vi "ChooseZones.vi"(8 "error in (no error)":errorcluster, 9 "NumberOfAttackers":i32, 10 "Game":refnum<class "Game.lvclass">, 11 "object in":refnum<class "Ally.lvclass">) -> (0 "error out":errorcluster, 2 "Zones":refnum<class "Zone.lvclass">[](array[class]), 3 "object out":refnum<class "Ally.lvclass">)   [LabVIEW 2023, in "Ally.lvclass"]
uses:
  Ally.lvclass
  Game_class/Game.lvclass
  Zone_class/Zone.lvclass
  Ally.lvclass/Ally.ctl
  Game_class/Game.lvclass/Game.ctl
  Parameters_class/Parameters.lvclass/Parameters.ctl
  Zone_class/zones.ctl
  Game_class/Read FieldRef.vi
  Game_class/Read NewParameters.vi
  Game_class/Read Parameters.lvclass.vi
  Parameters_class/Read AttakingOurselves.vi
  Field_class/Field.lvclass
  Parameters_class/Parameters.lvclass
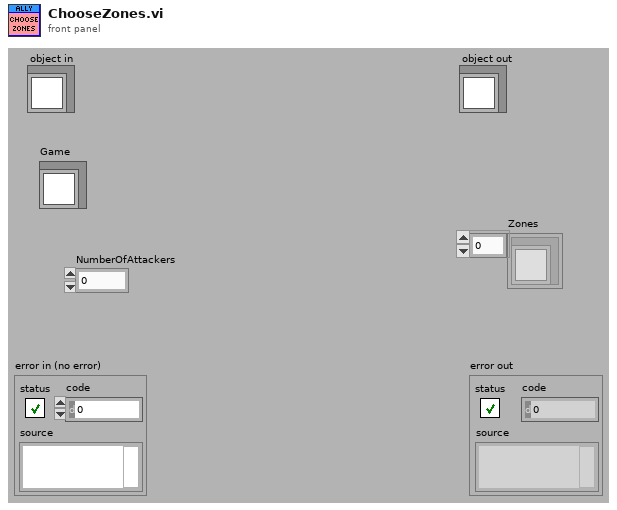
[diagram p1: front panel]
types:
  T1 = typedef "NewParameters.ctl" = cluster{"PenaltyDistance":dbl, "DistanceAttackerToBackBall":dbl, "Division":enum16{"Div B", "Div A"}, "DistanceToAvoidyEnemyRobot":dbl, "BallPlacementDistance":dbl, "DisatanceBehindBallToStealBall":dbl, "MaxDistanceToPositionKickoff":dbl, "BlockEnemyTarget":bool, "MaxStopVAng":dbl, "DistanceMarkerToEnemy":dbl, "IgnoreDribblerContact":bool, "DistanceToBeginEnemyPosession":dbl, "GoToBallWhenEnemyNotMoving":bool, "EnemyDistanceToReduceVelocity":dbl, "TurnOnEnemyDistanceToReduceVelocity":bool, "EnemyDistanceToShootOutBall":dbl, "DefenseKickBall":bool, "MoreKickToGoal? (0-0.3)":dbl, "ChipKickInEnemyField":bool, "ShootOutRobotId":dbl, "FieldLenghtDenominatorInShootOut":dbl, "AdjustPositionInBallPlacement":bool, "PowerGodPass":dbl, "VelocityAbortEnemyPos":dbl, "MaxDistToBeginPass":dbl, "MinDistToBeginPass":dbl, "VelocityInDirects":dbl, "BadDribblerIDs":i32[], "NewKickToDistanceAroundBall":dbl, "PowerAvoidColisionMarker":dbl, "DistanceToAvoidColisionMarker":dbl, "AvoidBallKick":dbl, "DistanceTryKick":dbl, "SuicideKickDIstance":dbl, "AdjustFirstKickDistance":dbl, "AvoidAimLessKick":dbl, "DistanceToAvoidyEnemyShootRobot ":dbl, "NumberOfMarkers":dbl, "PotField":bool, "PIDLateral":bool, "MinDistanceFirstKickX":dbl, "MinDistanceFirstKickY":dbl, "FractionOfDistToTouchGround\nAfterChipKick":dbl, "FractionOfKickxWhen\nComposedWithKickz":dbl, "Style":T2, "MoveInTurnState":bool, "DistFromEnemyToConsider\nMoveInTurnState":dbl, "CascadePID":bool, "TurnAroundParameters":cluster{"Radius":dbl, "Multiplier":dbl, "ChordAngle":dbl}, "SafeDriveVel":dbl, "DistanceToGoToBackBall":dbl, "minDistanceToNotFinish\nEnemyPossession":dbl, "OneTouchShot":cluster{"angleFactor":dbl, "maxAngle":dbl, "Attack":bool, "Defense":bool}, "OpenAngleToGoal":cluster{"minAngle":dbl, "maxAngle":dbl, "minEvaluation":dbl}, "ShotInterception":cluster{"shotSpeed":dbl, "minEnemySpeed":dbl, "maxEnemySpeed":dbl, "minEvaluation":dbl}, "AllyTeamArray":T3[], "maxDefendersNumber":i32, "Zone":cluster{"GuardPositionArray":dbl[][], "ZoneMidField":dbl[], "CenterForwardWidth":dbl}, "MinEvaluationToShoot":dbl, "PassInterception":cluster{"maxPassSpeed":dbl, "minPassSpeed":dbl, "minEnemySpeed":dbl, "chipPassDistance":dbl, "chipPassEvaluation":dbl, "minEvaluation":dbl, "maxEnemySpeed":dbl}, "PassDistance":cluster{"maxDistance":dbl, "minDistance":dbl}, "receiverSpeed":dbl, "maxBallSpeed":dbl, "slackTime":dbl, "Turning radius":dbl, "Turning v_ang":dbl, "AlignError":cluster{"Distance":dbl, "Orientation":dbl, "V_norm(m/s)":dbl, "V_ang (rad/s)":dbl}, "RobotRadius":dbl, "KickerDistance":dbl, "keeper angle  to cover goalpost":dbl}
  T2 = typedef "Style.ctl" = enum16{"Insanity", "Offensive", "Defensive"}
  T3 = typedef "AllyTeam.ctl" = enum16{"Keeper", "Defender", "Attacker"}
  T4 = cluster{"GuardPositionArray":dbl[][], "ZoneMidField":dbl[], "CenterForwardWidth":dbl}
  T5 = typedef "Zone.lvclass/zones.ctl" = enum16{"Field", "LeftSide", "RightSide", "MidField", "LeftForward", "RightForward", "LeftMidField", "RightMidField", "LeftWing", "CenterForward", "RightWing", "Size"}
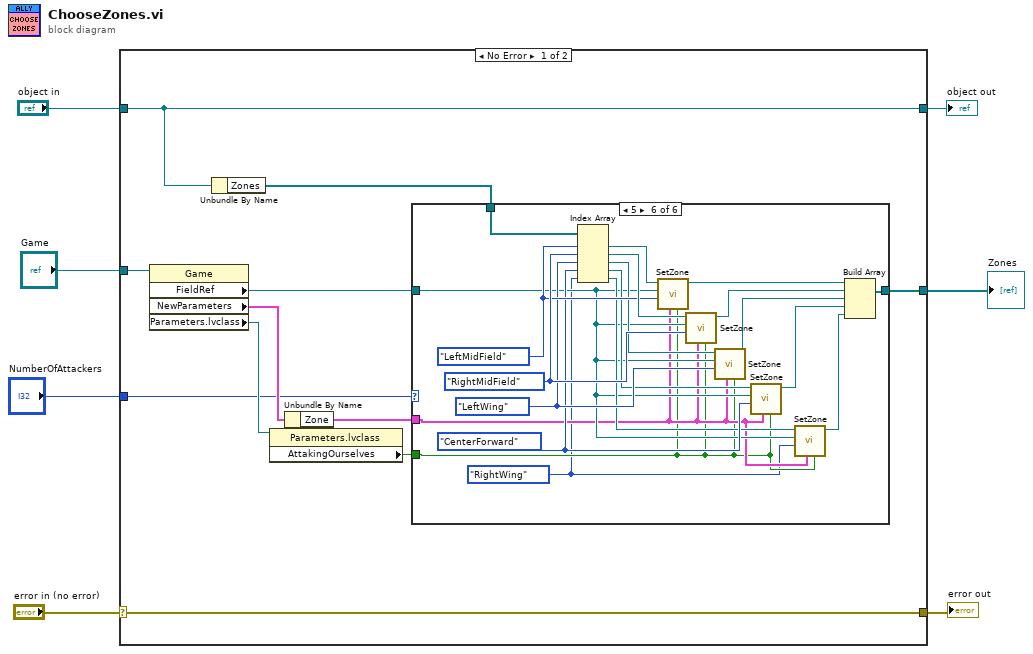
[diagram p0: block diagram]
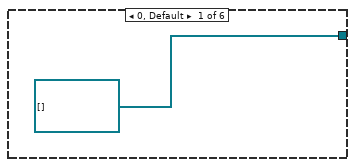
[diagram p2: hidden frame]
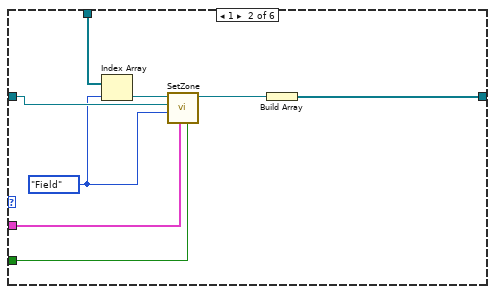
[diagram p3: hidden frame]
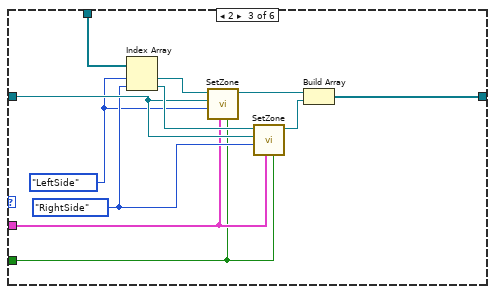
[diagram p4: hidden frame]
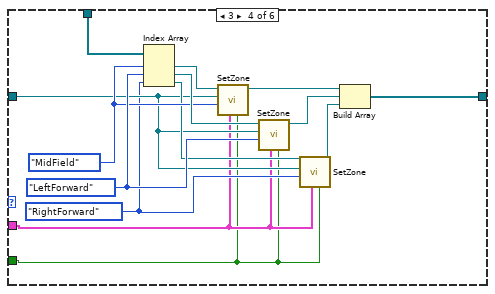
[diagram p5: hidden frame]
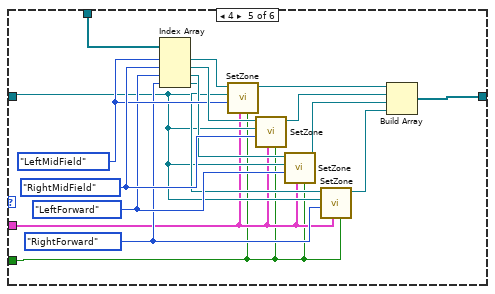
[diagram p6: hidden frame]
diagram:
  n1 = case shown="No Error" "error in (no error)" {
    selector: "error in (no error)" -> [w18 w91]
    tunnel: [w18 w91] -> w6
    tunnel: [w17 w90] -> w4
    tunnel: "object in" -> [w17 w90]
    tunnel: "Game" -> [w16 _]
    tunnel: "NumberOfAttackers" -> [w13 _]
    tunnel: [w12 _] -> w1
    frame No Error {
      n2 = property class="Game"(reference=w16) -> ("FieldRef"=w10:refnum<class "Field.lvclass">, "NewParameters"=w15:T1, "Parameters.lvclass"=w14:refnum<class "Parameters.lvclass">)  [unwired: 1 in, 2 out]
      n3 = Unbundle By Name(w17) -> ("Zones"=w11:refnum<class "Zone.lvclass">[])
      n4 = property class="Parameters.lvclass"(reference=w14) -> ("AttakingOurselves"=w8:bool)  [unwired: 1 in, 2 out]
      n5 = Unbundle By Name(w15) -> ("Zone"=w9:T4)
      n6 = case shown="5" w13 {
        tunnel: [refnum<class "Zone.lvclass">[] [] ("Array") w21 w28 w39 w59 w76] -> w12
        tunnel: w11 -> [_ w26 w36 w46 w60 w77]
        tunnel: w10 -> [_ w25 w34 w44 w55 w74]
        tunnel: w9 -> [_ w24 w31 w42 w54 w73]
        tunnel: w8 -> [_ w23 w30 w41 w53 w72]
        frame 0, Default {
        }
        frame 1 {
          w20 = zones."Field" ("Enum")
          n7 = Index Array(array=w26, index=w20) -> (element=w27:refnum<class "Zone.lvclass">)
          n8 = call "SetZone.vi"("AttackingOurselves"=w23, "ZoneParameters"=w24, "Enum"=w20, "Field"=w25, "object in"=w27) -> ("object out"=w22:refnum<class "Zone.lvclass">)  [unwired: 5 in, 1 out]
          n9 = Build Array(w22) -> (w21:refnum<class "Zone.lvclass">[])
        }
        frame 2 {
          w32 = zones."LeftSide" ("Enum")
          w33 = zones."RightSide" ("Enum")
          n10 = Index Array(array=w36, index #1=w32, index #2=w33) -> (element #1=w37:refnum<class "Zone.lvclass">, element #2=w35:refnum<class "Zone.lvclass">)
          n11 = call "SetZone.vi"("AttackingOurselves"=w30, "ZoneParameters"=w31, "Enum"=w32, "Field"=w34, "object in"=w37) -> ("object out"=w38:refnum<class "Zone.lvclass">)  [unwired: 5 in, 1 out]
          n12 = call "SetZone.vi"("AttackingOurselves"=w30, "ZoneParameters"=w31, "Enum"=w33, "Field"=w34, "object in"=w35) -> ("object out"=w29:refnum<class "Zone.lvclass">)  [unwired: 5 in, 1 out]
          n13 = Build Array(w38, w29) -> (w28:refnum<class "Zone.lvclass">[])
        }
        frame 3 {
          w43 = zones."RightForward" ("Enum")
          w48 = zones."MidField" ("Enum")
          w49 = zones."LeftForward" ("Enum")
          n14 = Index Array(array=w46, index #1=w48, index #2=w49, index #3=w43) -> (element #1=w51:refnum<class "Zone.lvclass">, element #2=w50:refnum<class "Zone.lvclass">, element #3=w45:refnum<class "Zone.lvclass">)
          n15 = call "SetZone.vi"("AttackingOurselves"=w41, "ZoneParameters"=w42, "Enum"=w48, "Field"=w44, "object in"=w51) -> ("object out"=w52:refnum<class "Zone.lvclass">)  [unwired: 5 in, 1 out]
          n16 = call "SetZone.vi"("AttackingOurselves"=w41, "ZoneParameters"=w42, "Enum"=w49, "Field"=w44, "object in"=w50) -> ("object out"=w47:refnum<class "Zone.lvclass">)  [unwired: 5 in, 1 out]
          n17 = call "SetZone.vi"("AttackingOurselves"=w41, "ZoneParameters"=w42, "Enum"=w43, "Field"=w44, "object in"=w45) -> ("object out"=w40:refnum<class "Zone.lvclass">)  [unwired: 5 in, 1 out]
          n18 = Build Array(w52, w47, w40) -> (w39:refnum<class "Zone.lvclass">[])
        }
        frame 4 {
          w56 = zones."RightForward" ("Enum")
          w62 = zones."LeftForward" ("Enum")
          w65 = zones."LeftMidField" ("Enum")
          w66 = zones."RightMidField" ("Enum")
          n19 = Index Array(array=w60, index #1=w65, index #2=w66, index #3=w62, index #4=w56) -> (element #1=w68:refnum<class "Zone.lvclass">, element #2=w67:refnum<class "Zone.lvclass">, element #3=w63:refnum<class "Zone.lvclass">, element #4=w57:refnum<class "Zone.lvclass">)
          n20 = call "SetZone.vi"("AttackingOurselves"=w53, "ZoneParameters"=w54, "Enum"=w65, "Field"=w55, "object in"=w68) -> ("object out"=w69:refnum<class "Zone.lvclass">)  [unwired: 5 in, 1 out]
          n21 = call "SetZone.vi"("AttackingOurselves"=w53, "ZoneParameters"=w54, "Enum"=w66, "Field"=w55, "object in"=w67) -> ("object out"=w64:refnum<class "Zone.lvclass">)  [unwired: 5 in, 1 out]
          n22 = call "SetZone.vi"("AttackingOurselves"=w53, "ZoneParameters"=w54, "Enum"=w62, "Field"=w55, "object in"=w63) -> ("object out"=w61:refnum<class "Zone.lvclass">)  [unwired: 5 in, 1 out]
          n23 = call "SetZone.vi"("AttackingOurselves"=w53, "ZoneParameters"=w54, "Enum"=w56, "Field"=w55, "object in"=w57) -> ("object out"=w58:refnum<class "Zone.lvclass">)  [unwired: 5 in, 1 out]
          n24 = Build Array(w69, w64, w61, w58) -> (w59:refnum<class "Zone.lvclass">[])
        }
        frame 5 {
          w70 = zones."RightWing" ("Enum")
          w78 = zones."CenterForward" ("Enum")
          w82 = zones."LeftWing" ("Enum")
          w85 = zones."LeftMidField" ("Enum")
          w86 = zones."RightMidField" ("Enum")
          n25 = Index Array(array=w77, index #1=w85, index #2=w86, index #3=w82, index #4=w78, index #5=w70) -> (element #1=w88:refnum<class "Zone.lvclass">, element #2=w87:refnum<class "Zone.lvclass">, element #3=w83:refnum<class "Zone.lvclass">, element #4=w79:refnum<class "Zone.lvclass">, element #5=w75:refnum<class "Zone.lvclass">)
          n26 = call "SetZone.vi"("AttackingOurselves"=w72, "ZoneParameters"=w73, "Enum"=w85, "Field"=w74, "object in"=w88) -> ("object out"=w89:refnum<class "Zone.lvclass">)  [unwired: 5 in, 1 out]
          n27 = call "SetZone.vi"("AttackingOurselves"=w72, "ZoneParameters"=w73, "Enum"=w86, "Field"=w74, "object in"=w87) -> ("object out"=w84:refnum<class "Zone.lvclass">)  [unwired: 5 in, 1 out]
          n28 = call "SetZone.vi"("AttackingOurselves"=w72, "ZoneParameters"=w73, "Enum"=w82, "Field"=w74, "object in"=w83) -> ("object out"=w81:refnum<class "Zone.lvclass">)  [unwired: 5 in, 1 out]
          n29 = call "SetZone.vi"("AttackingOurselves"=w72, "ZoneParameters"=w73, "Enum"=w78, "Field"=w74, "object in"=w79) -> ("object out"=w80:refnum<class "Zone.lvclass">)  [unwired: 5 in, 1 out]
          n30 = call "SetZone.vi"("AttackingOurselves"=w72, "ZoneParameters"=w73, "Enum"=w70, "Field"=w74, "object in"=w75) -> ("object out"=w71:refnum<class "Zone.lvclass">)  [unwired: 5 in, 1 out]
          n31 = Build Array(w89, w84, w81, w80, w71) -> (w76:refnum<class "Zone.lvclass">[])
        }
      }
    }
    frame Error {
    }
  }
  "error out" <- w6
  "object out" <- w4
  "Zones" <- w1
